vi "calculator.vi"() -> ()   [LabVIEW 2025]
panel:
  in  "Enum":T1(ring)
  out "String 3":string
  in  "String 2":string
  in  "String2":string
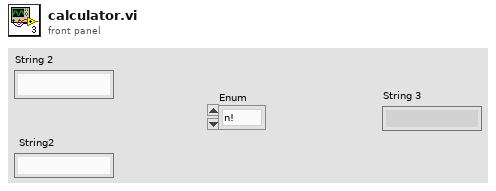
[diagram p1: front panel]
types:
  T1 = enum16{"n!", "sqrt", "^2", "+", "-", "*", "cos", "sin", "exp", "/"}
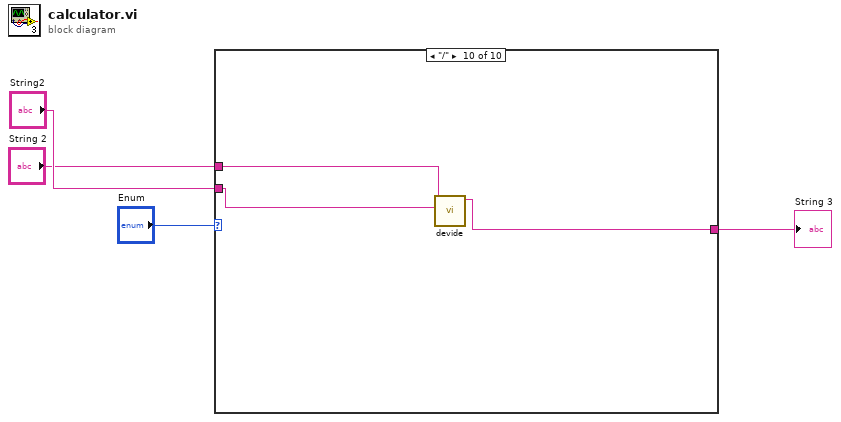
[diagram p0: block diagram]
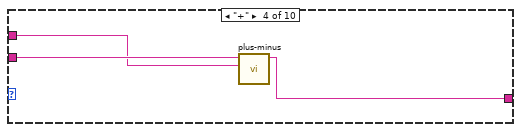
[diagram p5: hidden frame]
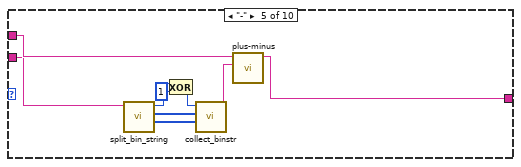
[diagram p6: hidden frame]
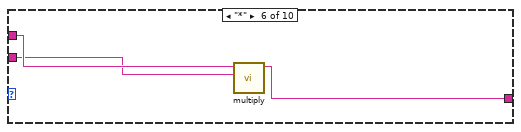
[diagram p7: hidden frame]
diagram:
  n1 = case shown="\"/\"" "Enum" {
    tunnel: "String2" -> [_ _ _ w7 w15 w18 _ _ _ w21]
    tunnel: "String 2" -> [_ _ _ w6 w16 w19 _ _ _ w22]
    tunnel: [_ _ _ w5 w8 w17 _ _ _ w20] -> w1
    frame "n!", Default {
    }
    frame "sqrt" {
    }
    frame "^2" {
    }
    frame "+" {
      n2 = call "plus-minus.vi"("String 2"=w6, "String"=w7) -> ("String 3"=w5:string)  [unwired: 9 in]
    }
    frame "-" {
      n3 = call "split_bin_string.vi"("String"=w15) -> ("Fraction"=w13:u8[], "Integer"=w14:u8[], "Sign"=w12:u8)  [unwired: 8 in]
      n4 = Exclusive Or(1:u8 1 ("y"), 2:w12) -> (0:w10:u8)
      n5 = call "collect_binstr.vi"("Fraction"=w13, "Integer"=w14, "Sign"=w10) -> ("String"=w9:string)  [unwired: 8 in]
      n6 = call "plus-minus.vi"("String 2"=w9, "String"=w16) -> ("String 3"=w8:string)  [unwired: 9 in]
    }
    frame "*" {
      n7 = call "multiply.vi"("String 2"=w18, "String"=w19) -> ("String 3"=w17:string)  [unwired: 9 in]
    }
    frame "cos" {
    }
    frame "sin" {
    }
    frame "exp" {
    }
    frame "/" {
      n8 = call "devide.vi"("String 2"=w21, "String"=w22) -> ("String 3"=w20:string)  [unwired: 9 in]
    }
  }
  "String 3" <- w1
